vi "THz Test controller.vi"() -> ()   [LabVIEW 2018, in "THz source modeule.lvlib"]
uses:
  THz source modeule.lvlib
  Messenger service/MessengerLib.lvlib
  ctl/THz Message for module.ctl
  ctl/THz commands enum.ctl
  ctl/VDI config constants.ctl
  ctl/THz sweep parameters.ctl
  ctl/Synth configs.ctl
panel:
  in  "Sweep parameters":T1={"Start [GHz]"=9.0, "End [GHz] "=9.0, "Rate [GHz/s]"=0.0, "Intermidiate [MHz]"=0.0, "Enable trigger"=FALSE} {"End [GHz]" min=9.0 max=15.0; "Intermidiate [MHz]" min=0.0 max=250.0; "Start [GHz]" min=9.0 max=15.0}
  out "Logger":string[](array[string])
  in  "VDI config constants":T2={"Master"={"Lower limit [GHz]"=8.0, "Upper limit [GHz]"=20.0, "Name"="VDIS0122", "Handle"=507261176, "Description"="VDI Synth"}, "Follower"={"Lower limit [GHz]"=0.0, "Upper limit [GHz]"=20.0, "Name"="VDIYT7", "Handle"=507251944, "Description"="VDI Tracking"}}
  in  "Disconnect":bool
  in  "Set parameters":bool
  in  "Connect":bool
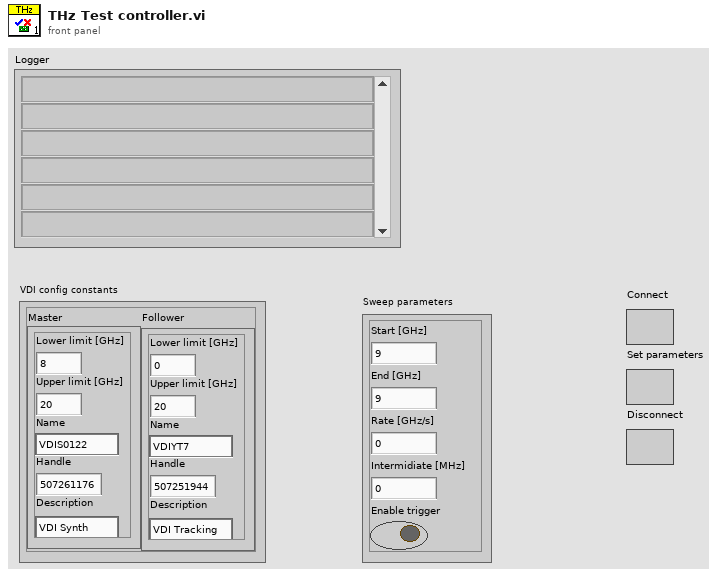
[diagram p1: front panel]
types:
  T1 = typedef "THz source modeule.lvlib/THz sweep parameters.ctl" = cluster{"Start [GHz]":dbl, "End [GHz] ":dbl, "Rate [GHz/s]":dbl, "Intermidiate [MHz]":dbl, "Enable trigger":bool}
  T2 = typedef "VDI config constants.ctl" = cluster{"Master":T3, "Follower":T3}
  T3 = typedef "THz source modeule.lvlib/Synth configs.ctl" = cluster{"Lower limit [GHz]":dbl, "Upper limit [GHz]":dbl, "Name":string, "Handle":u32, "Description":string}
  T4 = enum8{"Enabled", "Disabled", "Disabled and Grayed Out"}
  T5 = typedef "THz source modeule.lvlib/THz Message for module.ctl" = cluster{"Command":T6, "Data":variant}
  T6 = typedef "THz source modeule.lvlib/THz commands enum.ctl" = enum16{"Ignore", "Initialize", "Update", "Set parameters", "Disconnect", "End"}
  T7 = typedef "MessengerLib.lvlib/MSG to TOP.ctl" = cluster{"Module":T8, "Response":string, "Data":variant, "Time":timestamp}
  T8 = typedef "Module name.ctl" = enum16{"Emty", "Magnet", "VTI", "Excitation", "Servo", "Acquisition", "Rotator", "Digitizer", "SMU2450", "Carousel", "Multimeter", "Tmp monitor", "Power monitor"}
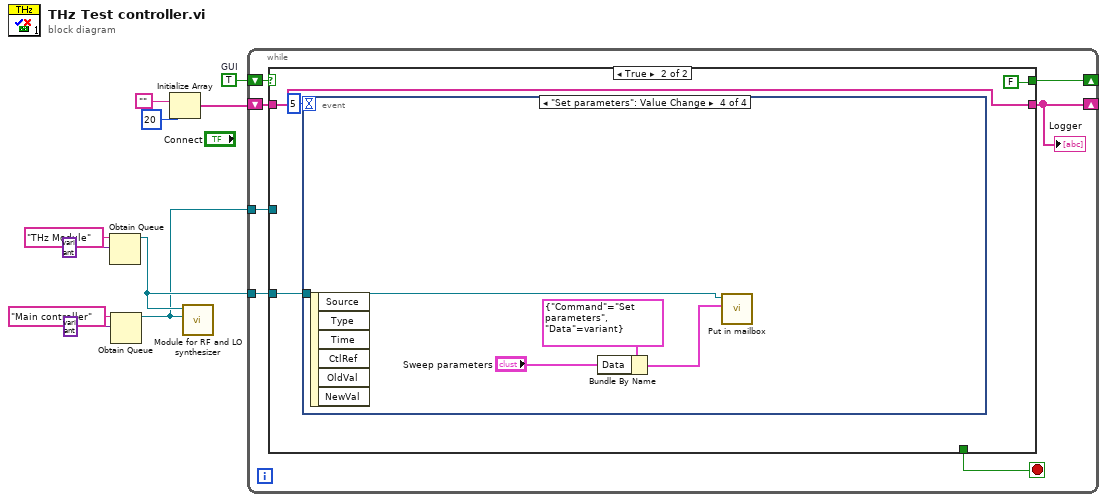
[diagram p0: block diagram]
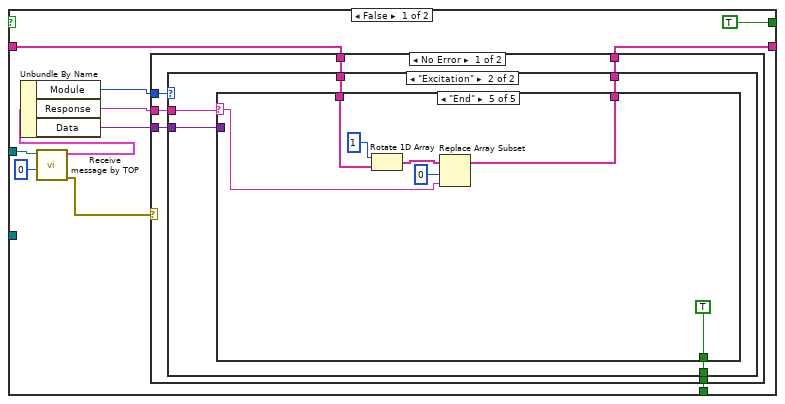
[diagram p2: hidden frame]
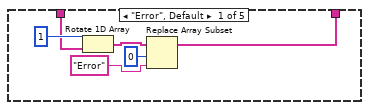
[diagram p4: hidden frame]
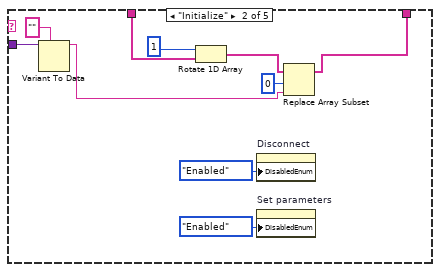
[diagram p5: hidden frame]
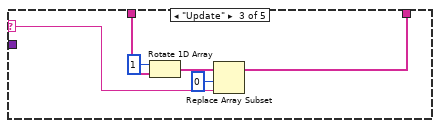
[diagram p6: hidden frame]
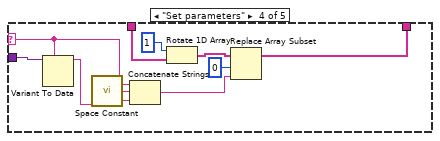
[diagram p7: hidden frame]
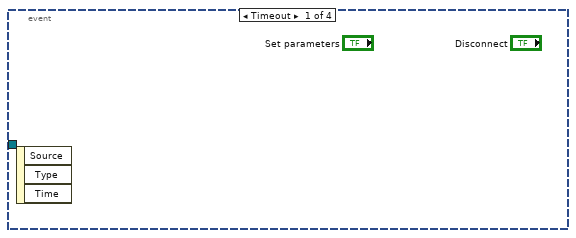
[diagram p9: hidden frame]
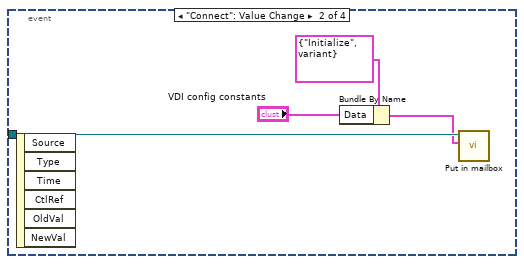
[diagram p10: hidden frame]
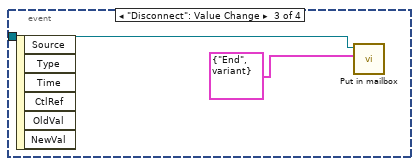
[diagram p11: hidden frame]
diagram:
  w10 = TRUE  # GUI
  n1 = Obtain Queue(name (unnamed)="THz Module", element data type=variant) -> (queue out=w5:refnum<queue>)  [unwired: 3 in, 2 out]
  n2 = Obtain Queue(name (unnamed)="Main controller", element data type=variant) -> (queue out=w4:refnum<queue>)  [unwired: 3 in, 2 out]
  n3 = Initialize Array("", 20 ("dimension size")) -> (w3:string[])
  n4 = call "Module for RF and LO synthesizer.vi"("Main controller mailbox"=w4, "THz module mailbox"=w5) -> ()  [unwired: 10 in]
  n5 = while {
    shift-right: [w16] -> _
    shift-left: w10 -> [w17]
    tunnel: w4 -> [w15]
    tunnel: w5 -> [w14]
    shift-right: [w11] -> _
    shift-left: w3 -> [w13]
    stop <- w12 stop-if-true
    n6 = case shown="True" w17 {
      tunnel: [TRUE FALSE] -> w16
      tunnel: w15 -> [w26 _]
      tunnel: w14 -> [_ w82]
      tunnel: w13 -> [w21 w81]
      tunnel: [w20 w81] -> w11
      tunnel: [w19 _] -> w12
      frame False {
        n7 = call "Receive message by TOP.vi"("timeout (100)"=0 ("timeout (-1)"), "Mailbox in"=w26) -> ("error out"=w18:errorcluster, "MSG packet"=w25:T7)  [unwired: 6 in, 2 out]
        n8 = Unbundle By Name(w25) -> ("Module"=w24:T8, "Response"=w23:string, "Data"=w22:variant)
        n9 = case shown="No Error" w18 {
          tunnel: w24 -> [w34 _]
          tunnel: w23 -> [w33 _]
          tunnel: w22 -> [w32 _]
          tunnel: w21 -> [w31 w80]
          tunnel: [w30 w80] -> w20
          tunnel: [w29 _] -> w19
          frame No Error {
            n10 = case shown="\"Excitation\"" w34 {
              tunnel: w33 -> [_ w40]
              tunnel: w32 -> [_ w39]
              tunnel: w31 -> [w35 w38]
              tunnel: [w35 w37] -> w30
              tunnel: [_ w36] -> w29
              frame "Emty", Default {
              }
              frame "Excitation" {
                n11 = case shown="\"End\"" w40 {
                  selector: w40 -> [_ _ w58 w66 w76]
                  tunnel: w39 -> [_ w56 _ w67 _]
                  tunnel: w38 -> [w42 w53 w60 w69 w74]
                  tunnel: [w43 w50 w57 w68 w73] -> w37
                  tunnel: [_ _ _ _ TRUE] -> w36
                  frame "Error", Default {
                    n12 = Rotate 1D Array(1:w42, 2:1 ("n")) -> (0:w46:string[])
                    n13 = Replace Array Subset(array=w46, new element="Error" ("new element/subarray"), index=0) -> (w43:string[])
                  }
                  frame "Initialize" {
                    n14 = Variant To Data(type="", Variant=w56) -> (data=w49:string)  [unwired: 1 in, 1 out]
                    n15 = Rotate 1D Array(1:w53, 2:1 ("n")) -> (0:w51:string[])
                    n16 = property on="Disconnect" class="Bool (strict)"("DisabledEnum"=T4."Enabled" ("Disabled")) -> ()  [unwired: 2 in, 2 out]
                    n17 = property on="Set parameters" class="Bool (strict)"("DisabledEnum"=T4."Enabled" ("Disabled")) -> ()  [unwired: 2 in, 2 out]
                    n18 = Replace Array Subset(array=w51, new element=w49, index=0) -> (w50:string[])
                  }
                  frame "Update" {
                    n19 = Rotate 1D Array(1:w60, 2:1 ("n")) -> (0:w62:string[])
                    n20 = Replace Array Subset(array=w62, new element=w58, index=0) -> (w57:string[])
                  }
                  frame "Set parameters" {
                    n21 = Variant To Data(type=w66, Variant=w67) -> (data=w64:string)  [unwired: 1 in, 1 out]
                    n22 = call <vilib>:"Space Constant.vi"() -> ("String"=w63:string)
                    n23 = Concatenate Strings(w66, w63, w64) -> (w65:string)
                    n24 = Rotate 1D Array(1:w69, 2:1 ("n")) -> (0:w72:string[])
                    n25 = Replace Array Subset(array=w72, new element=w65, index=0) -> (w68:string[])
                  }
                  frame "End" {
                    n26 = Rotate 1D Array(1:w74, 2:1 ("n")) -> (0:w78:string[])
                    n27 = Replace Array Subset(array=w78, new element=w76, index=0) -> (w73:string[])
                  }
                }
              }
            }
          }
          frame Error {
          }
        }
      }
      frame True {
        n28 = event shown="[3] \"Set parameters\": Value Change" {
          selector: _ -> [_ _ _ _]
          dyn-events: _ -> [_ _ _ _]
          timeout: 5 ("milliseconds to wait") -> [_ _ _ _]
          tunnel: w82 -> [_ w86 w89 w91]
          event Timeout {
            n29 = event-data() -> ()  [unwired: 1 in, 3 out]
          }
          event "Connect": Value Change {
            n30 = event-data() -> ()  [unwired: 1 in, 6 out]
            n31 = Bundle By Name(cluster=T5 {"Command"=enum."Initialize", "Data"=variant} ("Incoming msg"), "Data"="VDI config constants") -> (w85:T5)
            n32 = call "Put in mailbox.vi"("Message"=w85, "Queue in"=w86) -> ()  [unwired: 7 in, 3 out]
          }
          event "Disconnect": Value Change {
            n33 = event-data() -> ()  [unwired: 1 in, 6 out]
            n34 = call "Put in mailbox.vi"("Message"=T5 {"Command"=enum."End", "Data"=variant} ("Incoming msg"), "Queue in"=w89) -> ()  [unwired: 7 in, 3 out]
          }
          event "Set parameters": Value Change {
            n35 = event-data() -> ()  [unwired: 1 in, 6 out]
            n36 = Bundle By Name(cluster=T5 {"Command"=enum."Set parameters", "Data"=variant} ("Incoming msg"), "Data"="Sweep parameters") -> (w93:T5)
            n37 = call "Put in mailbox.vi"("Message"=w93, "Queue in"=w91) -> ()  [unwired: 7 in, 3 out]
          }
        }
      }
    }
    "Logger" <- w11
  }
